vi "oax_Cursor Run.vi"(8 "error in (no error)":errorcluster, 9 "millisecond multiple":u32, 11 "Order waveform":refnum<vi>) -> (0 "error out":errorcluster)   [LabVIEW 2017]
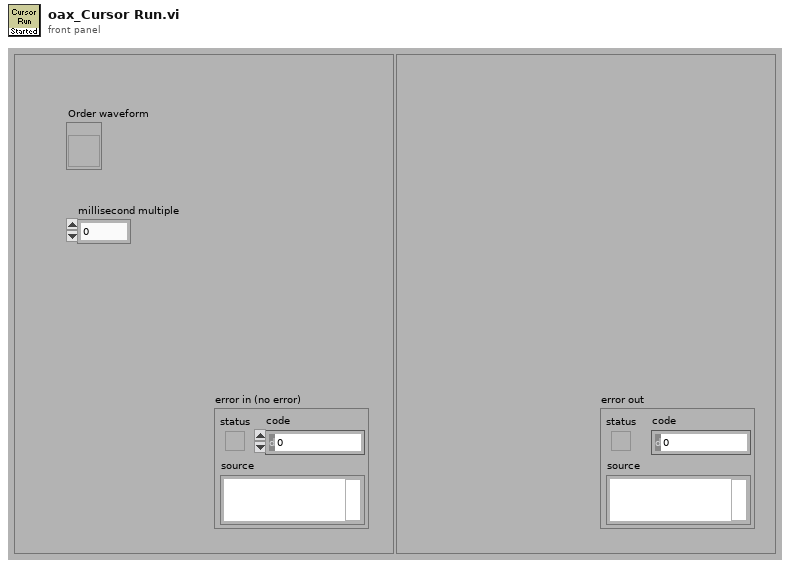
[diagram p1: front panel]
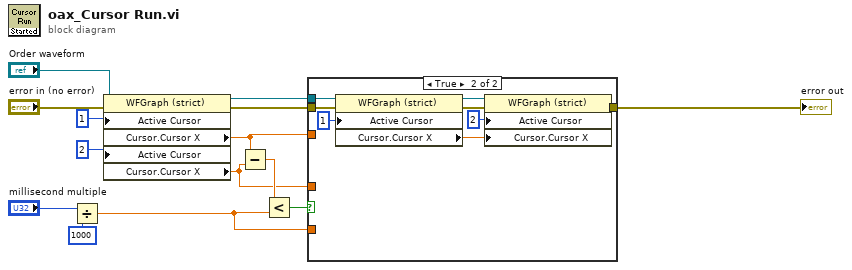
[diagram p0: block diagram]
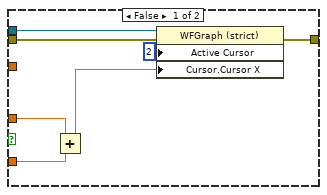
[diagram p2: hidden frame]
diagram:
  n1 = Divide(x="millisecond multiple", y=u32 1000) -> (x/y=w3:dbl)
  n2 = property on="Property Node" class="WFGraph (strict)"(reference="Order waveform", error in="error in (no error)", "Active Cursor"=u32 1, "Active Cursor"=u32 2) -> (reference out=w5:refnum<vi>, error out=w4:errorcluster, "Cursor.Cursor X"=w2:dbl, "Cursor.Cursor X"=w1:dbl)
  n3 = Subtract(x=w2, y=w1) -> (x-y=w7:dbl)
  n4 = Less?(x=w7, y=w3) -> (x < y?=w6:bool)
  n5 = case shown="True" w6 {
    tunnel: w5 -> [w20 w29]
    tunnel: w4 -> [w19 w28]
    tunnel: [w16 w22] -> w10
    tunnel: w3 -> [w18 _]
    tunnel: w2 -> [_ _]
    tunnel: w1 -> [w15 _]
    frame False {
      n6 = Add(x=w15, y=w18) -> (x+y=w17:dbl)
      n7 = property on="Property Node" class="WFGraph (strict)"(reference=w20, error in=w19, "Active Cursor"=u32 2, "Cursor.Cursor X"=w17) -> (error out=w16:errorcluster)  [unwired: 1 out]
    }
    frame True {
      n8 = property on="Property Node" class="WFGraph (strict)"(reference=w29, error in=w28, "Active Cursor"=u32 1) -> (reference out=w26:refnum<vi>, error out=w25:errorcluster, "Cursor.Cursor X"=w23:dbl)
      n9 = property on="Property Node" class="WFGraph (strict)"(reference=w26, error in=w25, "Active Cursor"=u32 2, "Cursor.Cursor X"=w23) -> (error out=w22:errorcluster)  [unwired: 1 out]
    }
  }
  "error out" <- w10
